vi "FindAddress.vi"() -> ()   [LabVIEW 2022 SP3]
uses:
  usb_relay_device/usb_relay_device.lvlib
panel:
  out "LastDigItt":string
  out "Relay Identifier":i32
  in  "Stop":bool
  out "serial_number":string
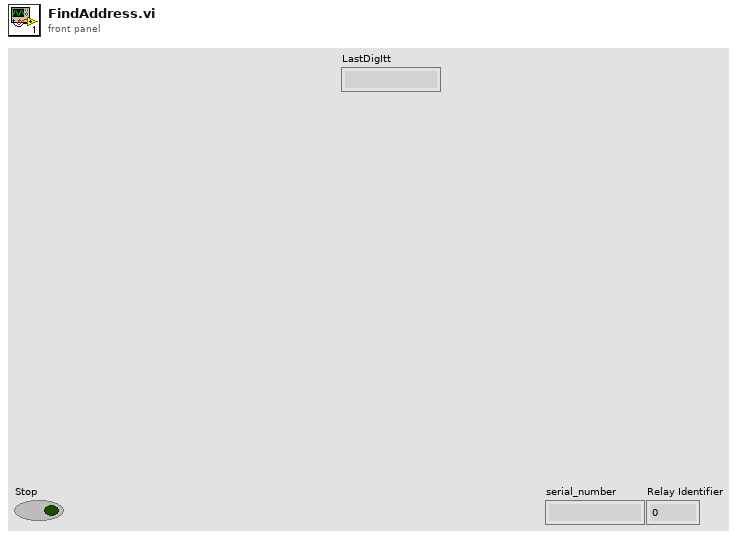
[diagram p1: front panel]
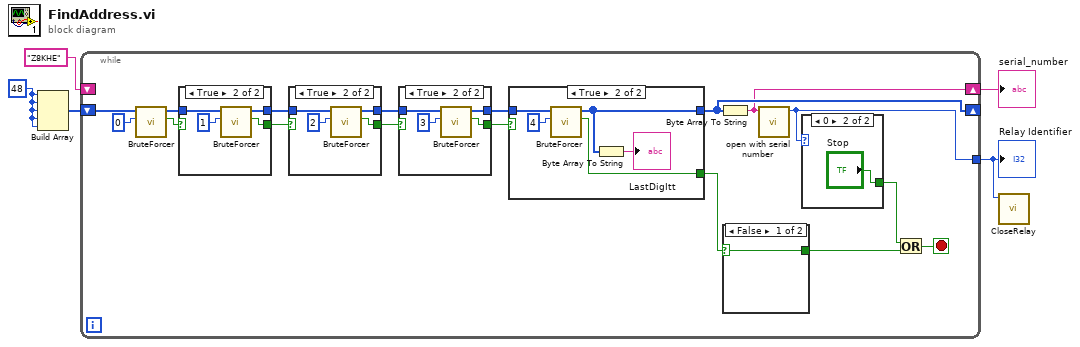
[diagram p0: block diagram]
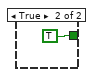
[diagram p2: hidden frame]
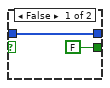
[diagram p3: hidden frame]
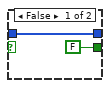
[diagram p4: hidden frame]
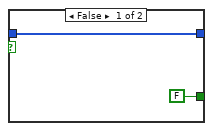
[diagram p5: hidden frame]
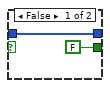
[diagram p6: hidden frame]
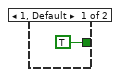
[diagram p7: hidden frame]
diagram:
  w1 = u8 48
  n1 = Build Array(w1, w1, w1, w1, w1) -> (w2:u8[])
  n2 = while {
    shift-right: [w9] -> w4
    shift-left: "Z8KHE" ("serial_number") -> [_]
    shift-right: [w10] -> _
    shift-left: w2 -> [w21]
    tunnel: [w22] -> w3
    stop <- w8 stop-if-true
    n3 = call "BruteForcer.vi"("Index"=0, "Array in"=w21) -> ("Rolled Over?"=w6:bool, "Array out"=w19:u8[])  [unwired: 8 in]
    n4 = case shown="True" w6 {
      tunnel: w19 -> [w45 w49]
      tunnel: [w45 w48] -> w12
      tunnel: [FALSE w47] -> w11
      frame False {
      }
      frame True {
        n5 = call "BruteForcer.vi"("Index"=1, "Array in"=w49) -> ("Rolled Over?"=w47:bool, "Array out"=w48:u8[])  [unwired: 8 in]
      }
    }
    n6 = case shown="True" w11 {
      tunnel: w12 -> [w26 w27]
      tunnel: [w26 w29] -> w18
      tunnel: [FALSE w30] -> w16
      frame False {
      }
      frame True {
        n7 = call "BruteForcer.vi"("Index"=2, "Array in"=w27) -> ("Rolled Over?"=w30:bool, "Array out"=w29:u8[])  [unwired: 8 in]
      }
    }
    n8 = case shown="True" w16 {
      tunnel: w18 -> [w32 w36]
      tunnel: [w32 w35] -> w17
      tunnel: [FALSE w34] -> w15
      frame False {
      }
      frame True {
        n9 = call "BruteForcer.vi"("Index"=3, "Array in"=w36) -> ("Rolled Over?"=w34:bool, "Array out"=w35:u8[])  [unwired: 8 in]
      }
    }
    n10 = case shown="True" w15 {
      tunnel: w17 -> [w38 w43]
      tunnel: [w38 w40] -> w10
      tunnel: [FALSE w42] -> w14
      frame False {
      }
      frame True {
        n11 = call "BruteForcer.vi"("Index"=4, "Array in"=w43) -> ("Rolled Over?"=w42:bool, "Array out"=w40:u8[])  [unwired: 8 in]
        n12 = Byte Array To String(unsigned byte array=w40) -> (string=→"LastDigItt":string)
      }
    }
    n13 = Byte Array To String(unsigned byte array=w10) -> (string=w9:string)
    n14 = case shown="False" w14 {
      selector: w14 -> [w23 _]
      tunnel: [w23 TRUE] -> w13
      frame False {
      }
      frame True {
      }
    }
    n15 = call "open with serial number.vi"("serial_number"=w9) -> ("Relay Identifier"=w22:i32)  [unwired: 9 in, 1 out]
    n16 = case shown="0" w22 {
      tunnel: [TRUE "Stop"] -> w7
      frame 1, Default {
      }
      frame 0 {
      }
    }
    n17 = Or(x=w7, y=w13) -> (x .or. y?=w8:bool)
  }
  "serial_number" <- w4
  "Relay Identifier" <- w3
  n18 = call "CloseRelay.vi"("Relay Identifier"=w3) -> ()  [unwired: 10 in, 1 out]
